vi "Accelerometer.vi"() -> ()   [LabVIEW 2010]
uses:
  <vilib>/eio/EIONode/EIONode.xnode
panel:
  in  "Acceleration Threshold":fxp<+/-,24,4> format="%.22g"
  in  "Fan Speed Control":fxp<+/-,20,5> format="%_6g"
  in  "Stop":bool
  in  "Sample Period (us)":u32
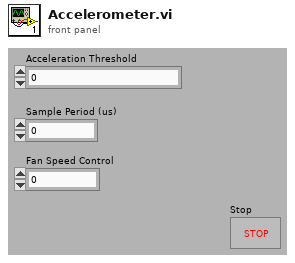
[diagram p1: front panel]
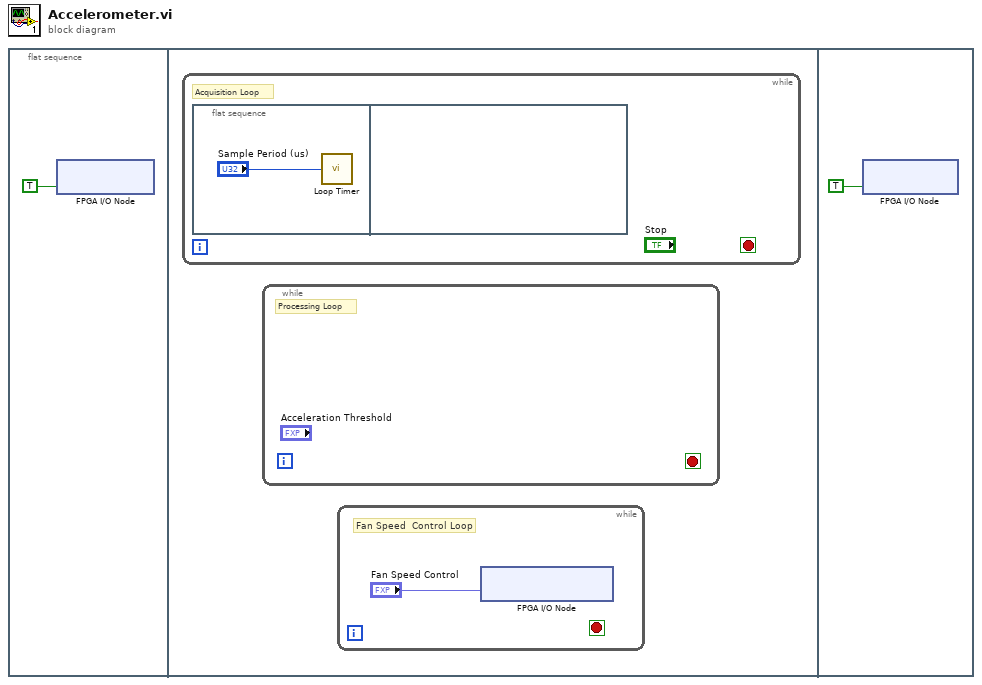
[diagram p0: block diagram]
diagram:
  n1 = flat-sequence {
    frame #0 {
      n2 = xnode "FPGA I/O Node"("Mod2/Start"=TRUE) -> ()  [unwired: 1 in, 1 out]
    }
    frame #1 {
      n3 = while {
        stop <- _ stop-if-true
        # "Acquisition Loop"
        n4 = flat-sequence {
          frame #0 {
            n5 = call "Loop Timer"("Count(uSec)"="Sample Period (us)") -> ()  [unwired: 1 out]
          }
          frame #1 {
          }
        }
      }
      n6 = while {
        stop <- _ stop-if-true
        # "Processing Loop"
      }
      n7 = while {
        stop <- _ stop-if-true
        # "Fan Speed  Control Loop"
        n8 = xnode "FPGA I/O Node"("Fan Speed Control"="Fan Speed Control") -> ()  [unwired: 1 in, 1 out]
      }
    }
    frame #2 {
      n9 = xnode "FPGA I/O Node"("Mod2/Stop"=TRUE ("Mod2/Start")) -> ()  [unwired: 1 in, 1 out]
    }
  }
